vi "Query Amplitude Mode.vi"(8 "error in (no error)":errorcluster, 11 "VISA resource name":refnum<visa-resource-name>) -> (0 "error out":errorcluster, 2 "Amplitude Mode":enum16{"Fixed", "Stepped Sweep", "List Sweep"}(ring), 3 "VISA resource name out":refnum<visa-resource-name>)   [LabVIEW 2017, in "Agilent PSG MXG Series.lvlib"]
uses:
  Agilent PSG MXG Series.lvlib
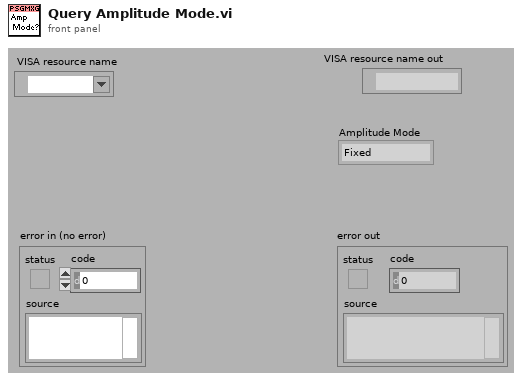
[diagram p1: front panel]
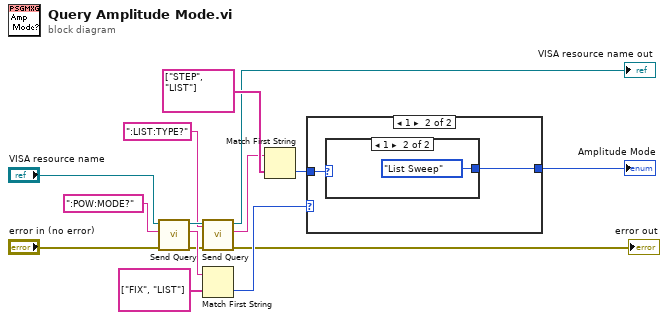
[diagram p0: block diagram]
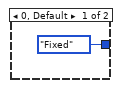
[diagram p2: hidden frame]
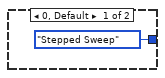
[diagram p3: hidden frame]
diagram:
  n1 = call "Send Query.vi"("error in (no error)"="error in (no error)", "write buffer"=":POW:MODE?", "VISA resource name"="VISA resource name") -> ("error out"=w7:errorcluster, "read buffer"=w10:string, "VISA resource name out"=w9:refnum<visa-resource-name>)  [unwired: 6 out]
  n2 = call "Send Query.vi"("error in (no error)"=w7, "write buffer"=":LIST:TYPE?", "VISA resource name"=w9) -> ("error out"=→"error out":errorcluster, "read buffer"=w6:string, "VISA resource name out"=→"VISA resource name out":refnum<visa-resource-name>)  [unwired: 6 out]
  n3 = Match First String(2:string[] ["FIX", "LIST"], 3:w10) -> (0:w5:i32)  [unwired: 1 out]
  n4 = Match First String(2:string[] ["STEP", "LIST"], 3:w6) -> (0:w4:i32)  [unwired: 1 out]
  n5 = case shown="1" w5 {
    tunnel: w4 -> [_ w18]
    tunnel: [enum16{"Fixed", "Stepped Sweep", "List Sweep"}."Fixed" ("Amplitude Mode") w17] -> w3
    frame 0, Default {
    }
    frame 1 {
      n6 = case shown="1" w18 {
        tunnel: [enum16{"Fixed", "Stepped Sweep", "List Sweep"}."Stepped Sweep" ("Amplitude Mode") enum16{"Fixed", "Stepped Sweep", "List Sweep"}."List Sweep" ("Amplitude Mode")] -> w17
        frame 0, Default {
        }
        frame 1 {
        }
      }
    }
  }
  "Amplitude Mode" <- w3
